vi "get str without last.vi"(11 "string":string) -> (3 "substring":string)   [LabVIEW 2019, in "SubVI.lvlib"]
uses:
  SubVI.lvlib
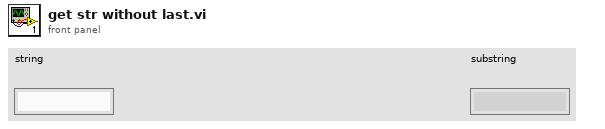
[diagram p1: front panel]
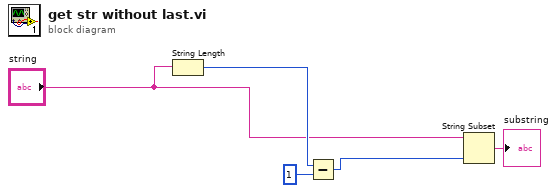
[diagram p0: block diagram]
diagram:
  n1 = String Length(string="string") -> (length=w5:i32)
  n2 = Subtract(x=w5, y=1) -> (x-y=w2:i32)
  n3 = String Subset(string="string", length (rest)=w2) -> (substring=→"substring":string)  [unwired: 1 in]
